vi "Mutex Set Priority Ceiling.vi"(8 "error in (no error)":errorcluster, 10 "priority ceiling":i32, 11 "Mutex in":T1) -> (0 "error out":errorcluster, 2 "old priority ceiling":i32, 3 "Mutex out":T1)   [LabVIEW 2013, in "POSIX Threads.lvlib" / "Mutex.lvclass"]
uses:
  Mutex.lvclass
  Controls/reference.ctl
  POSIX Thread Object/POSIX Thread Object.lvclass/POSIX Thread Object.ctl
  POSIX Thread Object/Private VIs/libpthread path.vi
  POSIX Thread Object/Private VIs/get pthread error.vi
  POSIX Thread Object/POSIX Thread Object.lvclass
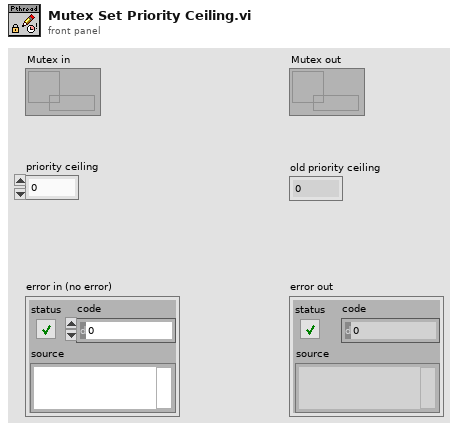
[diagram p1: front panel]
types:
  T1 = typedef "POSIX Threads.lvlib/Mutex.lvclass/reference.ctl" = refnum<data-value>
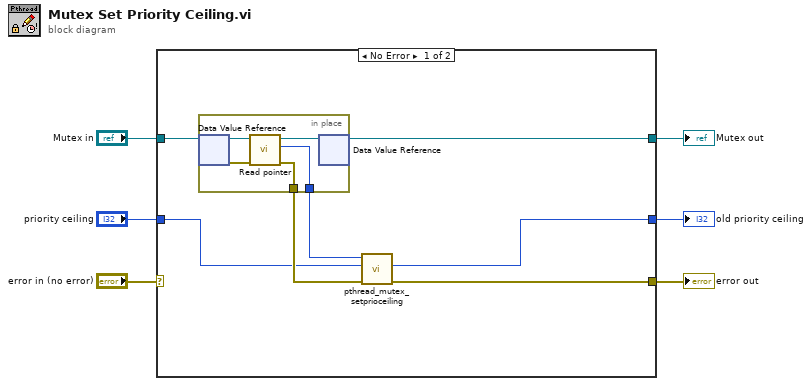
[diagram p0: block diagram]
diagram:
  n1 = case shown="No Error" "error in (no error)" {
    selector: "error in (no error)" -> [_ w20]
    tunnel: [w10 w20] -> w5
    tunnel: "Mutex in" -> [w13 w19]
    tunnel: [w12 w19] -> w3
    tunnel: "priority ceiling" -> [w8 _]
    tunnel: [w7 _] -> w1
    frame No Error {
      n2 = in-place {
        in-place-border: [w15] -> w11
        in-place-border: [w14] -> w9
        n3 = in-place-dvr #1(w13) -> (w18:refnum<class "Mutex.lvclass">, w16:errorcluster)
        n4 = call "Read pointer.vi"("error in (no error)"=w16, "POSIX Thread Object in"=w18) -> ("error out"=w15:errorcluster, "pointer"=w14:u64, "POSIX Thread Object out"=w17:refnum<class "Mutex.lvclass">)  [unwired: 7 in]
        n5 = in-place-dvr #1(w17) -> (w12:T1)  [unwired: 1 out]
      }
      n6 = call "pthread_mutex_setprioceiling.vi"("error in (no error)"=w11, "priority ceiling"=w8, "mutex ptr in"=w9) -> ("error out"=w10:errorcluster, "old priority ceiling"=w7:i32)  [unwired: 6 in, 1 out]
    }
    frame Error {
    }
  }
  "Mutex out" <- w3
  "error out" <- w5
  "old priority ceiling" <- w1
